vi "Is Class Data Control.vi"(8 "error in (no error)":errorcluster, 10 "Item Name":string, 11 "Path":path) -> (0 "error out":errorcluster, 3 "Is Class Data Control?":bool)   [LabVIEW 2023]
doc: "Checks to see if <B>Item Name</B> is a class data for control for the possible class identified by <B>Path</B>."
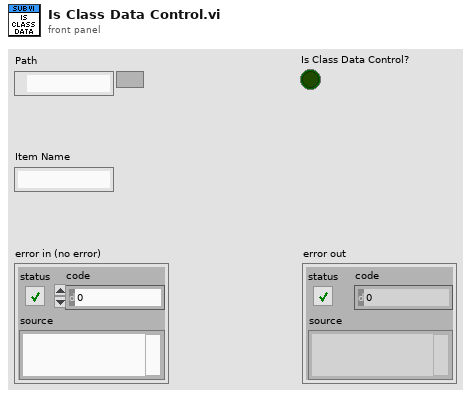
[diagram p1: front panel]
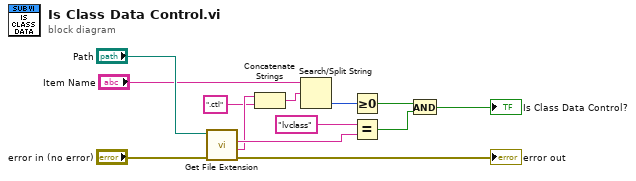
[diagram p0: block diagram]
diagram:
  n1 = call <vilib>:"Get File Extension.vi"("error in (no error)"="error in (no error)", "file"="Path") -> ("error out"=→"error out":errorcluster, "filename without extension"=w6:string, "lowercase file extension"=w10:string)  [unwired: 5 in, 2 out]
  n2 = Concatenate Strings(w6, ".ctl" ("string")) -> (w4:string)
  n3 = Search/Split String(string="Item Name", search string/char (-)=w4) -> (offset of match=w2:i32)  [unwired: 1 in, 2 out]
  n4 = Greater Or Equal To 0?(x=w2) -> (x >= 0?=w1:bool)
  n5 = Equal?(x="lvclass" ("y"), y=w10) -> (x = y?=w8:bool)
  n6 = And(x=w1, y=w8) -> (x .and. y?=→"Is Class Data Control?":bool)
